vi "Close Body References.vi"(8 "error in (no error)":errorcluster, 11 "BodyData":T1={"ClippedEdges"=0, "HandLeftConfidence"=1, "HandLeftState"=1, "HandRightConfidence"=1, "HandRightState"=1, "IsRestricted"=FALSE, "IsTracked"=FALSE, "JointOrientations"=refnum, "Joints"=refnum, "Lean"=refnum, "LeanTrackingState"=0, "TrackingId"=0} {"LeanTrackingState" items=["NotTracked", "Inferred", "Tracked"]; "HandRightState" items=["Unknown", "NotTracked", "Open", "Closed", "Lasso"]; "HandRightConfidence" items=["Low", "High"]; "HandLeftState" items=["Unknown", "NotTracked", "Open", "Closed", "Lasso"]; "HandLeftConfidence" items=["Low", "High"]; "ClippedEdges" items=["None"=0, "Right"=1, "Left"=2, "Top"=4, "Bottom"=8]}) -> (0 "error out":errorcluster)   [LabVIEW 2014]
uses:
  Type Defs/BodyData.ctl
  Microsoft.Kinect
  LVH-KinectOne.lvlib
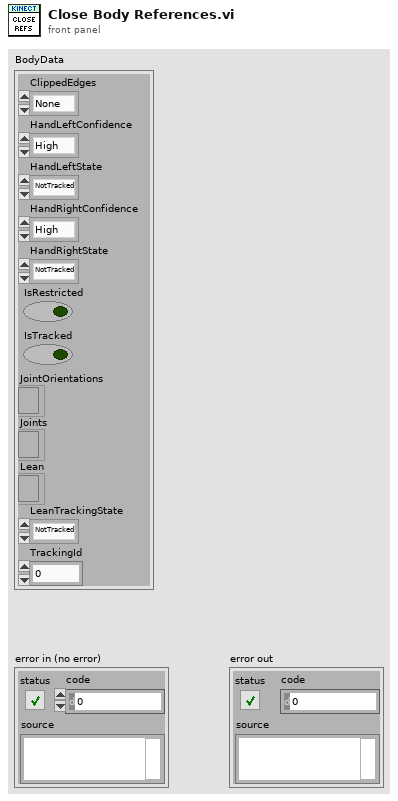
[diagram p1: front panel]
types:
  T1 = typedef "LVH-KinectOne.lvlib/BodyData.ctl" = cluster{"ClippedEdges":i32, "HandLeftConfidence":i32, "HandLeftState":i32, "HandRightConfidence":i32, "HandRightState":i32, "IsRestricted":bool, "IsTracked":bool, "JointOrientations":refnum<k24>, "Joints":refnum<k24>, "Lean":refnum<k24>, "LeanTrackingState":i32, "TrackingId":u64}
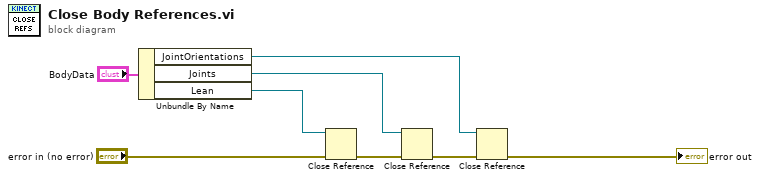
[diagram p0: block diagram]
diagram:
  n1 = Unbundle By Name("BodyData") -> ("JointOrientations"=w2:refnum<k24>, "Joints"=w3:refnum<k24>, "Lean"=w4:refnum<k24>)
  n2 = Close Reference(reference=w4, error in (no error)="error in (no error)") -> (error out=w7:errorcluster)
  n3 = Close Reference(reference=w3, error in (no error)=w7) -> (error out=w6:errorcluster)
  n4 = Close Reference(reference=w2, error in (no error)=w6) -> (error out=→"error out":errorcluster)
